vi "Func-엑셀 데이터를 그래프로 출력.vi"() -> ()   [LabVIEW 2015] (continued)
1252.26\n1252.28\n1252.29\n1252.31\n1252.33\n1252.34\n1252.36\n1252.38\n1252.39\n1252.41\n1252.43\n1252.44\n1252.46\n1252.48\n1252.49\n1252.51\n1252.53\n1252.54\n1252.56\n1252.58\n1252.59\n1252.61\n1252.63\n1252.64\n1252.66\n1252.68\n1252.69\n1252.71\n1252.73\n1252.74\n1252.76\n1252.78\n1252.79\n1252.81\n1252.83\n1252.84\n1252.86\n1252.88\n1252.89\n1252.91\n1252.93\n1252.94\n1252.96\n1252.98\n1252.99\n1253.01\n1253.03\n1253.04\n1253.06\n1253.08\n1253.09\n1253.11\n1253.13\n1253.14\n1253.16\n1253.18\n1253.2\n1253.21\n1253.23\n1253.24\n1253.26\n1253.28\n1253.3\n1253.31\n1253.33\n1253.34\n1253.36\n1253.38\n1253.39\n1253.41\n1253.43\n1253.44\n1253.46\n1253.48\n1253.49\n1253.51\n1253.53\n1253.55\n1253.56\n1253.58\n1253.59\n1253.61\n1253.63\n1253.64\n1253.66\n1253.68\n1253.69\n1253.71\n1253.73\n1253.74\n1253.76\n1253.78\n1253.79\n1253.81\n1253.83\n1253.84\n1253.86\n1253.88\n1253.9\n1253.91\n1253.93\n1253.94\n1253.96\n1253.98\n1253.99\n1254.01\n1254.03\n1254.04\n1254.06\n1254.08\n1254.09\n1254.11\n1254.13\n1254.14\n1254.16\n1254.18\n1254.19\n1254.21\n1254.23\n1254.25\n1254.26\n1254.28\n1254.29\n1254.31\n1254.33\n1254.35\n1254.36\n1254.38\n1254.39\n1254.41\n1254.43\n1254.44\n1254.46\n1254.48\n1254.5\n1254.51\n1254.53\n1254.54\n1254.56\n1254.58\n1254.59\n1254.61\n1254.63\n1254.64\n1254.66\n1254.68\n1254.69\n1254.71\n1254.73\n1254.74\n1254.76\n1254.78\n1254.79\n1254.81\n1254.83\n1254.84\n1254.86\n1254.88\n1254.89\n1254.91\n1254.93\n1254.94\n1254.96\n1254.98\n1254.99\n1255.01\n1255.03\n1255.04\n1255.06\n1255.08\n1255.09\n1255.11\n1255.13\n1255.15\n1255.16\n1255.18\n1255.19\n1255.21\n1255.23\n1255.24\n1255.26\n1255.28\n1255.29\n1255.31\n1255.33\n1255.34\n1255.36\n1255.38\n1255.39\n1255.41\n1255.43\n1255.44\n1255.46\n1255.48\n1255.49\n1255.51\n1255.53\n1255.54\n1255.56\n1255.58\n1255.59\n1255.61\n1255.63\n1255.64\n1255.66\n1255.68\n1255.69\n1255.71\n1255.73\n1255.74\n1255.76\n1255.78\n1255.79\n1255.81\n1255.83\n1255.84\n1255.86\n1255.88\n1255.89\n1255.91\n1255.93\n1255.95\n1255.96\n1255.98\n1255.99\n1256.01\n1256.03\n1256.04\n1256.06\n1256.08\n1256.09\n1256.11\n1256.13\n1256.14\n1256.16\n1256.18\n1256.19\n1256.21\n1256.23\n1256.24\n1256.26\n1256.28\n1256.3\n1256.31\n1256.33\n1256.34\n1256.36\n1256.38\n1256.39\n1256.41\n1256.43\n1256.44\n1256.46\n1256.48\n1256.49\n1256.51\n1256.53\n1256.54\n1256.56\n1256.58\n1256.59\n1256.61\n1256.63\n1256.65\n1256.66\n1256.68\n1256.69\n1256.71\n1256.73\n1256.74\n1256.76\n1256.78\n1256.79\n1256.81\n1256.83\n1256.85\n1256.86\n1256.88\n1256.9\n1256.91\n1256.93\n1256.94\n1256.96\n1256.98\n1257\n1257.01\n1257.03\n1257.04\n1257.06\n1257.08\n1257.09\n1257.11\n1257.13\n1257.14\n1257.16\n1257.18\n1257.2\n1257.21\n1257.23\n1257.25\n1257.26\n1257.28\n1257.29\n1257.31\n1257.33\n1257.35\n1257.36\n1257.38\n1257.39\n1257.41\n1257.43\n1257.45\n1257.46\n1257.48\n1257.49\n1257.51\n1257.53\n1257.54\n1257.56\n1257.58\n1257.6\n1257.61\n1257.63\n1257.64\n1257.66\n1257.68\n1257.69\n1257.71\n1257.73\n1257.74\n1257.76\n1257.78\n1257.79\n1257.81\n1257.83\n1257.84\n1257.86\n1257.88\n1257.89\n1257.91\n1257.93\n1257.94\n1257.96\n1257.98\n1257.99\n1258.01\n1258.03\n1258.04\n1258.06\n1258.08\n1258.09\n1258.11\n1258.13\n1258.14\n1258.16\n1258.18\n1258.19\n1258.21\n1258.23\n1258.24\n1258.26\n1258.28\n1258.29\n1258.31\n1258.33\n1258.35\n1258.36\n1258.38\n1258.39\n1258.41\n1258.43\n1258.44\n1258.46\n1258.48\n1258.49\n1258.51\n1258.53\n1258.54\n1258.56\n1258.58\n1258.59\n1258.61\n1258.63\n1258.64\n1258.66\n1258.68\n1258.69\n1258.71\n1258.73\n1258.74\n1258.76\n1258.78\n1258.79\n1258.81\n1258.83\n1258.85\n1258.86\n1258.88\n1258.89\n1258.91\n1258.93\n1258.94\n1258.96\n1258.98\n1258.99\n1259.01\n1259.03\n1259.05\n1259.06\n1259.08\n1259.09\n1259.11\n1259.13\n1259.14\n1259.16\n1259.18\n1259.19\n1259.21\n1259.23\n1259.24\n1259.26\n1259.28\n1259.3\n1259.31\n1259.33\n1259.34\n1259.36\n1259.38\n1259.4\n1259.41\n1259.43\n1259.44\n1259.46\n1259.48\n1259.49\n1259.51\n1259.53\n1259.54\n1259.56\n1259.58\n1259.59\n1259.61\n1259.63\n1259.65\n1259.66\n1259.68\n1259.69\n1259.71\n1259.73\n1259.75\n1259.76\n1259.78\n1259.8\n1259.81\n1259.83\n1259.85\n1259.86\n1259.88\n1259.89\n1259.91\n1259.93\n1259.94\n1259.96\n1259.98\n1260\n1260.01\n1260.03\n1260.04\n1260.06\n1260.08\n1260.09\n1260.11\n1260.13\n1260.14\n1260.16\n1260.18\n1260.19\n1260.21\n1260.23\n1260.24\n1260.26\n1260.28\n1260.29\n1260.31\n1260.33\n1260.34\n1260.36\n1260.38\n1260.39\n1260.41\n1260.43\n1260.44\n1260.46\n1260.48\n1260.49\n1260.51\n1260.53\n1260.54\n1260.56\n1260.58\n1260.59\n1260.61\n1260.63\n1260.65\n1260.66\n1260.68\n1260.69\n1260.71\n1260.73\n1260.74\n1260.76\n1260.78\n1260.79\n1260.81\n1260.83\n1260.84\n1260.86\n1260.88\n1260.89\n1260.91\n1260.93\n1260.94\n1260.96\n1260.98\n1260.99\n1261.01\n1261.03\n1261.04\n1261.06\n1261.08\n1261.09\n1261.11\n1261.13\n1261.14\n1261.16\n1261.18\n1261.19\n1261.21\n1261.23\n1261.24\n1261.26\n1261.28\n1261.29\n1261.31\n1261.33\n1261.34\n1261.36\n1261.38\n1261.39\n1261.41\n1261.43\n1261.44\n1261.46\n1261.48\n1261.49\n1261.51\n1261.53\n1261.54\n1261.56\n1261.58\n1261.59\n1261.61\n1261.63\n1261.64\n1261.66\n1261.68\n1261.69\n1261.71\n1261.73\n1261.74\n1261.76\n1261.78\n1261.79\n1261.81\n1261.83\n1261.84\n1261.86\n1261.88\n1261.89\n1261.91\n1261.93\n1261.94\n1261.96\n1261.98\n1261.99\n1262.01\n1262.03\n1262.05\n1262.06\n1262.08\n1262.09\n1262.11\n1262.13\n1262.15\n1262.16\n1262.18\n1262.19\n1262.21\n1262.23\n1262.24\n1262.26\n1262.28\n1262.29\n1262.31\n1262.33\n1262.34\n1262.36\n1262.38\n1262.39\n1262.41\n1262.43\n1262.44\n1262.46\n1262.48\n1262.5\n1262.51\n1262.53\n1262.55\n1262.56\n1262.58\n1262.6\n1262.61\n1262.63\n1262.64\n1262.66\n1262.68\n1262.69\n1262.71\n1262.73\n1262.75\n1262.76\n1262.78\n1262.79\n1262.81\n1262.83\n1262.85\n1262.86\n1262.88\n1262.89\n1262.91\n1262.93\n1262.94\n1262.96\n1262.98\n1262.99\n1263.01\n1263.03\n1263.04\n1263.06\n1263.08\n1263.1\n1263.11\n1263.13\n1263.14\n1263.16\n1263.18\n1263.19\n1263.21\n1263.23\n1263.24\n1263.26\n1263.28\n1263.29\n1263.31\n1263.33\n1263.35\n1263.36\n1263.38\n1263.39\n1263.41\n1263.43\n1263.45\n1263.46\n1263.48\n1263.5\n1263.51\n1263.53\n1263.54\n1263.56\n1263.58\n1263.59\n1263.61\n1263.63\n1263.64\n1263.66\n1263.68\n1263.69\n1263.71\n1263.73\n1263.74\n1263.76\n1263.78\n1263.79\n1263.81\n1263.83\n1263.84\n1263.86\n1263.88\n1263.89\n1263.91\n1263.93\n1263.94\n1263.96\n1263.98\n1263.99\n1264.01\n1264.03\n1264.04\n1264.06\n1264.08\n1264.09\n1264.11\n1264.13\n1264.14\n1264.16\n1264.18\n1264.19\n1264.21\n1264.23\n1264.24\n1264.26\n1264.28\n1264.29\n1264.31\n1264.33\n1264.34\n1264.36\n1264.38\n1264.39\n1264.41\n1264.43\n1264.44\n1264.46\n1264.48\n1264.49\n1264.51\n1264.53\n1264.55\n1264.56\n1264.58\n1264.59\n1264.61\n1264.63\n1264.64\n1264.66\n1264.68\n1264.69\n1264.71\n1264.73\n1264.74\n1264.76\n1264.78\n1264.79\n1264.81\n1264.83\n1264.84\n1264.86\n1264.88\n1264.89\n1264.91\n1264.93\n1264.94\n1264.96\n1264.98\n1264.99\n1265.01\n1265.03\n1265.04\n1265.06\n1265.08\n1265.09\n1265.11\n1265.13\n1265.14\n1265.16\n1265.18\n1265.19\n1265.21\n1265.23\n1265.25\n1265.26\n1265.28\n1265.29\n1265.31\n1265.33\n1265.34\n1265.36\n1265.38\n1265.39\n1265.41\n1265.43\n1265.44\n1265.46\n1265.48\n1265.5\n1265.51\n1265.53\n1265.54\n1265.56\n1265.58\n1265.6\n1265.61\n1265.63\n1265.64\n1265.66\n1265.68\n1265.69\n1265.71\n1265.73\n1265.75\n1265.76\n1265.78\n1265.79\n1265.81\n1265.83\n1265.85\n1265.86\n1265.88\n1265.89\n1265.91\n1265.93\n1265.95\n1265.96\n1265.98\n1265.99\n1266.01\n1266.03\n1266.04\n1266.06\n1266.08\n1266.09\n1266.11\n1266.13\n1266.14\n1266.16\n1266.18\n1266.19\n1266.21\n1283.85\n1283.86\n1283.9\n1283.93\n1283.96\n1284\n1284.03\n1284.06\n1284.1\n1284.13\n1284.16\n1284.2\n1284.23\n1284.26\n1284.3\n1284.33\n1284.36\n1284.4\n1284.43\n1284.46\n1284.49\n1284.53\n1284.56\n1284.59\n1284.63\n1284.66\n1284.7\n1284.73\n1284.76\n1284.8\n1284.83\n1284.86\n1284.9\n1284.93\n1284.96\n1284.99\n1285.03\n1285.06\n1285.09\n1285.13\n1285.16\n1285.2\n1285.23\n1285.26\n1285.3\n1285.33\n1285.36\n1285.4\n1285.43\n1285.46\n1285.5\n1285.53\n1285.56\n1285.6\n1285.63\n1285.66\n1285.7\n1285.73\n1285.76\n1285.79\n1285.83\n1285.86\n1285.9\n1285.93\n1285.96\n1286\n1286.03\n1286.06\n1286.1\n1286.13\n1286.16\n1286.2\n1286.23\n1286.26\n1286.3\n1286.33\n1286.36\n1286.4\n1286.43\n1286.46\n1286.5\n1286.53\n1286.56\n1286.6\n1286.63\n1286.66\n1286.7\n1286.73\n1286.76\n1286.8\n1286.83\n1286.86\n1286.9\n1286.93\n1286.96\n1287\n1287.03\n1287.06\n1287.1\n1287.13\n1287.16\n1287.2\n1287.23\n1287.26\n1287.3\n1287.33\n1287.36\n1287.39\n1287.43\n1287.46\n1287.49\n1287.53\n1287.56\n1287.59\n1287.63\n1287.66\n1287.71\n1287.73\n1287.76\n1287.8\n1287.83\n1287.86\n1287.9\n1287.93\n1287.96\n1288\n1288.03\n1288.06\n1288.09\n1288.13\n1288.16\n1288.19\n1288.23\n1288.26\n1288.3\n1288.33\n1288.36\n1288.4\n1288.43\n1288.46\n1288.5\n1288.53\n1288.56\n1288.6\n1288.63\n1288.66\n1288.7\n1288.73\n1288.76\n1288.8\n1288.83\n1288.86\n1288.89\n1288.93\n1288.96\n1289\n1289.03\n1289.06\n1289.1\n1289.13\n1289.16\n1289.2\n1289.23\n1289.26\n1289.3\n1289.33\n1289.36\n1289.4\n1289.43\n1289.46\n1289.5\n1289.53\n1289.56\n1289.6\n1289.63\n1289.66\n1289.7\n1289.73\n1289.76\n1289.8\n1289.83\n1289.86\n1289.9\n1289.93\n1289.96\n1290\n1290.03\n1290.06\n1290.1\n1290.13\n1290.16\n1290.2\n1290.23\n1290.26\n1290.3\n1290.33\n1290.36\n1290.39\n1290.43\n1290.46\n1290.49\n1290.53\n1290.56\n1290.6\n1290.63\n1290.66\n1290.69\n1290.75\n1290.76\n1290.8\n1290.83\n1290.86\n1290.9\n1290.93\n1290.96\n1291\n1291.03\n1291.06\n1291.1\n1291.13\n1291.16\n1291.19\n1291.23\n1291.26\n1291.29\n1291.35\n1291.36\n1291.4\n1291.43\n1291.46\n1291.5\n1291.53\n1291.56\n1291.6\n1291.63\n1291.66\n1291.7\n1291.73\n1291.76\n1291.8\n1291.83\n1291.86\n1291.9\n1291.95\n1291.96\n1292\n1292.03\n1292.06\n1292.1\n1292.13\n1292.16\n1292.2\n1292.23\n1292.26\n1292.3\n1292.33\n1292.36\n1292.4\n1292.43\n1292.46\n1292.5\n1292.55\n1292.56\n1292.6\n1292.63\n1292.66\n1292.7\n1292.73\n1292.76\n1292.8\n1292.83\n1292.86\n1292.9\n1292.93\n1292.96\n1293\n1293.03\n1293.06\n1293.1\n1293.15\n1293.16\n1293.2\n1293.23\n1293.26\n1293.3\n1293.33\n1293.36\n1293.4\n1293.43\n1293.46\n1293.49\n1293.53\n1293.56\n1293.6\n1293.63\n1293.66\n1293.71\n1293.73\n1293.76\n1293.8\n1293.83\n1293.86\n1293.9\n1293.93\n1293.96\n1294\n1294.03\n1294.06\n1294.1\n1294.13\n1294.16\n1294.2\n1294.23\n1294.26\n1294.29\n1294.33\n1294.36\n1294.39\n1294.43\n1294.46\n1294.5\n1294.53\n1294.56\n1294.6\n1294.63\n1294.66\n1294.7\n1294.73\n1294.76\n1294.8\n1294.83\n1294.86\n1294.9\n1294.95\n1294.96\n1294.99\n1295.03\n1295.06\n1295.1\n1295.13\n1295.16\n1295.2\n1295.23\n1295.26\n1295.3\n1295.33\n1295.36\n1295.4\n1295.43\n1295.46\n1295.5\n1295.53\n1295.58\n1295.61\n1295.63\n1295.66\n1295.7\n1295.73\n1295.76\n1295.8\n1295.83\n1295.86\n1295.9\n1295.93\n1295.96\n1296\n1296.03\n1296.06\n1296.1\n1296.13\n1296.18\n1296.2\n1296.23\n1296.26\n1296.3\n1296.33\n1296.36\n1296.4\n1296.43\n1296.46\n1296.5\n1296.53\n1296.56\n1296.6\n1296.63\n1296.66\n1296.7\n1296.73\n1296.76\n1296.81\n1296.83\n1296.86\n1296.89\n1296.93\n1296.96\n1297\n1297.03\n1297.06\n1297.1\n1297.13\n1297.16\n1297.2\n1297.23\n1297.26\n1297.3\n1297.33\n1297.36\n1297.39\n1297.43\n1297.46\n1297.49\n1297.53\n1297.56\n1297.6\n1297.63\n1297.66\n1297.7\n1297.73\n1297.76\n1297.8\n1297.83\n1297.86\n1297.9\n1297.93\n1297.98\n1298\n1298.03\n1298.06\n1298.1\n1298.13\n1298.16\n1298.2\n1298.23\n1298.26\n1298.3\n1298.33\n1298.36\n1298.4\n1298.43\n1298.46\n1298.5\n1298.53\n1298.56\n1298.61\n1298.65\n1298.66\n1298.7\n1298.73\n1298.76\n1298.8\n1298.83\n1298.86\n1298.9\n1298.93\n1298.96\n1299\n1299.03\n1299.06\n1299.1\n1299.13\n1299.16\n1299.2\n1299.23\n1299.26\n1299.3\n1299.33\n1299.36\n1299.4\n1299.43\n1299.46\n1299.5\n1299.53\n1299.56\n1299.6\n1299.63\n1299.66\n1299.7\n1299.73\n1299.76\n1299.79\n1299.85\n1299.86\n1299.89\n1299.93\n1299.96\n1300\n1300.03\n1300.06\n1300.1\n1300.13\n1300.16\n1300.2\n1300.23\n1300.26\n1300.3\n1300.33\n1300.36\n1300.41\n1300.43\n1300.46\n1300.49\n1300.53\n1300.56\n1300.6\n1300.63\n1300.66\n1300.7\n1300.73\n1300.77\n1300.78\n1300.79\n1300.79\n1300.8\n1300.81\n1300.82\n1300.83\n1300.84\n1300.84\n1300.85\n1300.86\n1300.87\n1300.88\n1300.89\n1300.89\n1300.9\n1300.91\n1300.92\n1300.93\n1300.94\n1300.94\n1300.95\n1300.96\n1300.97\n1300.98\n1300.99\n1300.99\n1301\n1301.01\n1301.02\n1301.03\n1301.04\n1301.04\n1301.05\n1301.06\n1301.07\n1301.08\n1301.09\n1301.09\n1301.1\n1301.11\n1301.12\n1301.13\n1301.14\n1301.14\n1301.15\n1301.16\n1301.17\n1301.18\n1301.19\n1301.19\n1301.2\n1301.21\n1301.22\n1301.23\n1301.24\n1301.24\n1301.25\n1301.26\n1301.27\n1301.28\n1301.29\n1301.29\n1301.3\n1301.31\n1301.32\n1301.33\n1301.34\n1301.34\n1301.35\n1301.36\n1301.37\n1301.38\n1301.39\n1301.39\n1301.4\n1301.41\n1301.42\n1301.43\n1301.44\n1301.44\n1301.45\n1301.46\n1301.47\n1301.48\n1301.49\n1301.49\n1301.5\n1301.51\n1301.52\n1301.53\n1301.54\n1301.55\n1301.55\n1301.56\n1301.57\n1301.58\n1301.59\n1301.59\n1301.6\n1301.61\n1301.62\n1301.63\n1301.64\n1301.64\n1301.65\n1301.66\n1301.67\n1301.68\n1301.69\n1301.69\n1301.7\n1301.71\n1301.72\n1301.73\n1301.74\n1301.74\n1301.75\n1301.76\n1301.77\n1301.78\n1301.79\n1301.79\n1301.8\n1301.81\n1301.82\n1301.83\n1301.84\n1301.84\n1301.85\n1301.86\n1301.87\n1301.88\n1301.89\n1301.9\n1301.9\n1301.91\n1301.92\n1301.93\n1301.94\n1301.94\n1301.95\n1301.96\n1301.97\n1301.98\n1301.99\n1302\n1302\n1302.01\n1302.02\n1302.03\n1302.04\n1302.04\n1302.05\n1302.06\n1302.07\n1302.08\n1302.09\n1302.09\n1302.1\n1302.11\n1302.12\n1302.13\n1302.14\n1302.15\n1302.15\n1302.16\n1302.17\n1302.18\n1302.19\n1302.19\n1302.2\n1302.21\n1302.22\n1302.23\n1302.24\n1302.25\n1302.25\n1302.26\n1302.27\n1302.28\n1302.29\n1302.29\n1302.3\n1302.31\n1302.32\n1302.33\n1302.34\n1302.35\n1302.35\n1302.36\n1302.37\n1302.38\n1302.39\n1302.39\n1302.4\n1302.41\n1302.42\n1302.43\n1302.44\n1302.44\n1302.45\n1302.46\n1302.47\n1302.48\n1302.49\n1302.5\n1302.5\n1302.51\n1302.52\n1302.53\n1302.54\n1302.54\n1302.55\n1302.56\n1302.57\n1302.58\n1302.59\n1302.6\n1302.6\n1302.61\n1302.62\n1302.63\n1302.64\n1302.64\n1302.65\n1302.66\n1302.67\n1302.68\n1302.69\n1302.7\n1302.7\n1302.71\n1302.72\n1302.73\n1302.74\n1302.74\n1302.75\n1302.76\n1302.77\n1302.78\n1302.79\n1302.79\n1302.8\n1302.81\n1302.82\n1302.83\n1302.84\n1302.84\n1302.85\n1302.86\n1302.87\n1302.88\n1302.89\n1302.89\n1302.9\n1302.91\n1302.92\n1302.93\n1302.94\n1302.94\n1302.95\n1302.96\n1302.97\n1302.98\n1302.99\n1302.99\n1303\n1303.01\n1303.02\n1303.03\n1303.04\n1303.04\n1303.05\n1303.06\n1303.07\n1303.08\n1303.09\n1303.09\n1303.1\n1303.11\n1303.12\n1303.13\n1303.14\n1303.14\n1303.15\n1303.16\n1303.17\n1303.18\n1303.19\n1303.19\n1303.2\n1303.21\n1303.22\n1303.23\n1303.24\n1303.24\n1303.25\n1303.26\n1303.27\n1303.28\n1303.29\n1303.29\n1303.3\n1303.31\n1303.32\n1303.33\n1303.34\n1303.34\n1303.35\n1303.36\n1303.37\n1303.38\n1303.39\n1303.39\n1303.4\n1303.41\n1303.42\n1303.43\n1303.44\n1303.44\n1303.45\n1303.46\n1303.47\n1303.48\n1303.49\n1303.49\n1303.5\n1303.51\n1303.52\n1303.53\n1303.54\n1303.54\n1303.55\n1303.56\n1303.57\n1303.58\n1303.59\n1303.59\n1303.6\n1303.61\n1303.62\n1303.63\n1303.64\n1303.64\n1303.65\n1303.66\n1303.67\n1303.68\n1303.69\n1303.69\n1303.7\n1303.71\n1303.72\n1303.73\n1303.74\n1303.74\n1303.75\n1303.76\n1303.77\n1303.78\n1303.79\n1303.79\n1303.8\n1303.81\n1303.82\n1303.83\n1303.84\n1303.84\n1303.85\n1303.86\n1303.87\n1303.88\n1303.89\n1303.89\n1303.9\n1303.91\n1303.92\n1303.93\n1303.94\n1303.94\n1303.95\n1303.96\n1303.97\n1303.98\n1303.99\n1303.99\n1304\n1304.01\n1304.02\n1304.03\n1304.04\n1304.04\n1304.05\n1304.06\n1304.07\n1304.08\n1304.09\n1304.09\n1304.1\n1304.11\n1304.12\n1304.13\n1304.14\n1304.14\n1304.15\n1304.16\n1304.17\n1304.18\n1304.19\n1304.19\n1304.2\n1304.21\n1304.22\n1304.23\n1304.24\n1304.24\n1304.25\n1304.26\n1304.27\n1304.28\n1304.29\n1304.3\n1304.3\n1304.31\n1304.32\n1304.33\n1304.34\n1304.34\n1304.35\n1304.36\n1304.37\n1304.38\n1304.39\n1304.39\n1304.4\n1304.41\n1304.42\n1304.43\n1304.44\n1304.44\n1304.45\n1304.46\n1304.47\n1304.48\n1304.49\n1304.49\n1304.5\n1304.51\n1304.52\n1304.53\n1304.54\n1304.54\n1304.55\n1304.56\n1304.57\n1304.58\n1304.59\n1304.59\n1304.6\n1304.61\n1304.62\n1304.63\n1304.64\n1304.64\n1304.65\n1304.66\n1304.67\n1304.68\n1304.69\n1304.69\n1304.7\n1304.71\n1304.72\n1304.73\n1304.74\n1304.74\n1304.75\n1304.76\n1304.77\n1304.78\n1304.79\n1304.79\n1304.8\n1304.81\n1304.82\n1304.83\n1304.84\n1304.84\n1304.85\n1304.86\n1304.87\n1304.88\n1304.89\n1304.89\n1304.9\n1304.91\n1304.92\n1304.93\n1304.94\n1304.94\n1304.95\n1304.96\n1304.97\n1304.98\n1304.99\n1305\n1305\n1305.01\n1305.02\n1305.03\n1305.04\n1305.04\n1305.05\n1305.06\n1305.07\n1305.08\n1305.09\n1305.09\n1305.1\n1305.11\n1305.12\n1305.13\n1305.14\n1305.14\n1305.15\n1305.16\n1305.17\n1305.18\n1305.19\n1305.19\n1305.2\n1305.21\n1305.22\n1305.23\n1305.24\n1305.25\n1305.25\n1305.26\n1305.27\n1305.28\n1305.29\n1305.29\n1305.3\n1305.31\n1305.32\n1305.33\n1305.34\n1305.35\n1305.35\n1305.36\n1305.37\n1305.38\n1305.39\n1305.39\n1305.4\n1305.41\n1305.42\n1305.43\n1305.44\n1305.44\n1305.45\n1305.46\n1305.47\n1305.48\n1305.49\n1305.49\n1305.5\n1305.51\n1305.52\n1305.53\n1305.54\n1305.54\n1305.55\n1305.56\n1305.57\n1305.58\n1305.59\n1305.6\n1305.6\n1305.61\n1305.62\n1305.63\n1305.64\n1305.64\n1305.65\n1305.66\n1305.67\n1305.68\n1305.69\n1305.7\n1305.7\n1305.71\n1305.72\n1305.73\n1305.74\n1305.74\n1305.75\n1305.77\n"
  in  "Y축 1":string="DPS 센서 전압(V)\n0.0003128\n0.00400914\n0.04822016\n0.09243478\n0.13661741\n0.18088003\n0.22513907\n0.26934129\n0.31354249\n0.35775453\n0.40194234\n0.44613013\n0.49034372\n0.53449279\n0.57871258\n0.62287194\n0.6670804\n0.71124184\n0.755328\n0.79956377\n0.84357244\n0.88760281\n0.93174618\n0.97576469\n1.01980484\n1.06384337\n1.10792947\n1.15197122\n1.19586015\n1.23986363\n1.28386247\n1.28381348\n1.24059355\n1.19588339\n1.15184271\n1.10791147\n1.06387436\n1.0198667\n0.97577345\n0.93180454\n0.88765496\n0.84360033\n0.79950494\n0.75538582\n0.71119487\n0.6671325\n0.62288386\n0.57876468\n0.53458673\n0.49045056\n0.44623077\n0.40202236\n0.35782215\n0.31363541\n0.26943782\n0.22521442\n0.18101114\n0.13677071\n0.09252615\n0.048247\n0.00409276\n0.00031384\n"
  # "엑셀 데이터를 그래프로 출력한다\n>> 열헤더 문자열 포함. (첫 라인)"
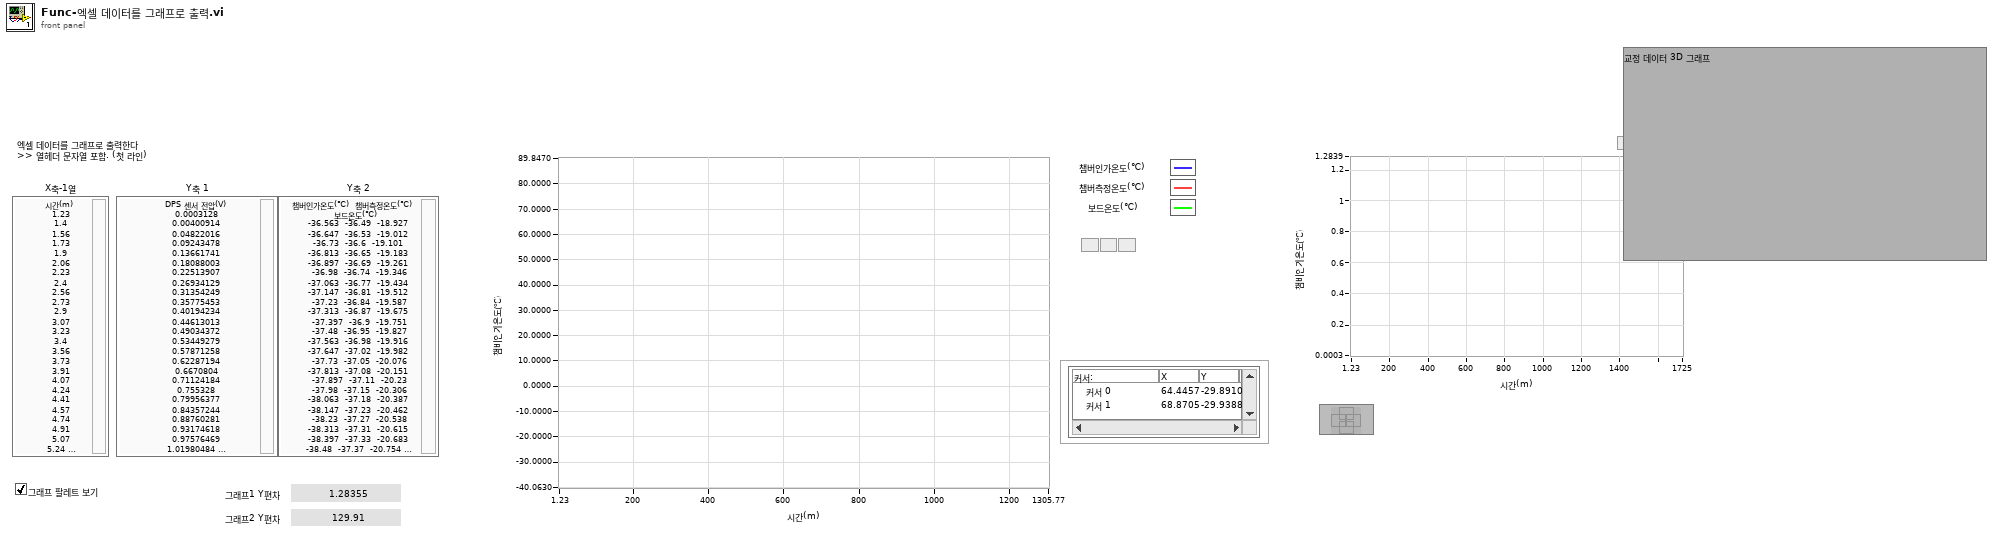
[diagram p1: front panel]
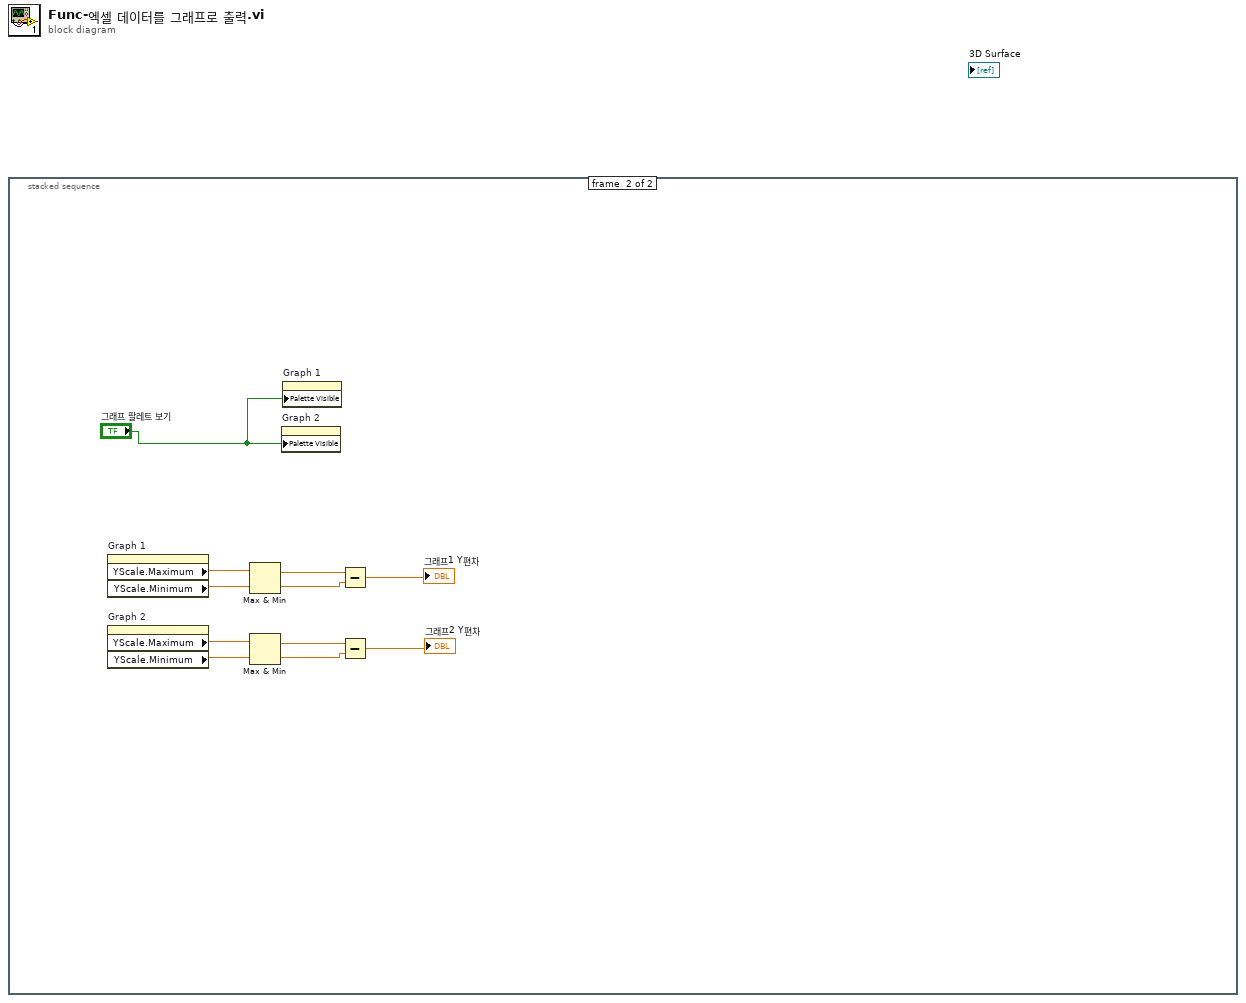
[diagram p0: block diagram]
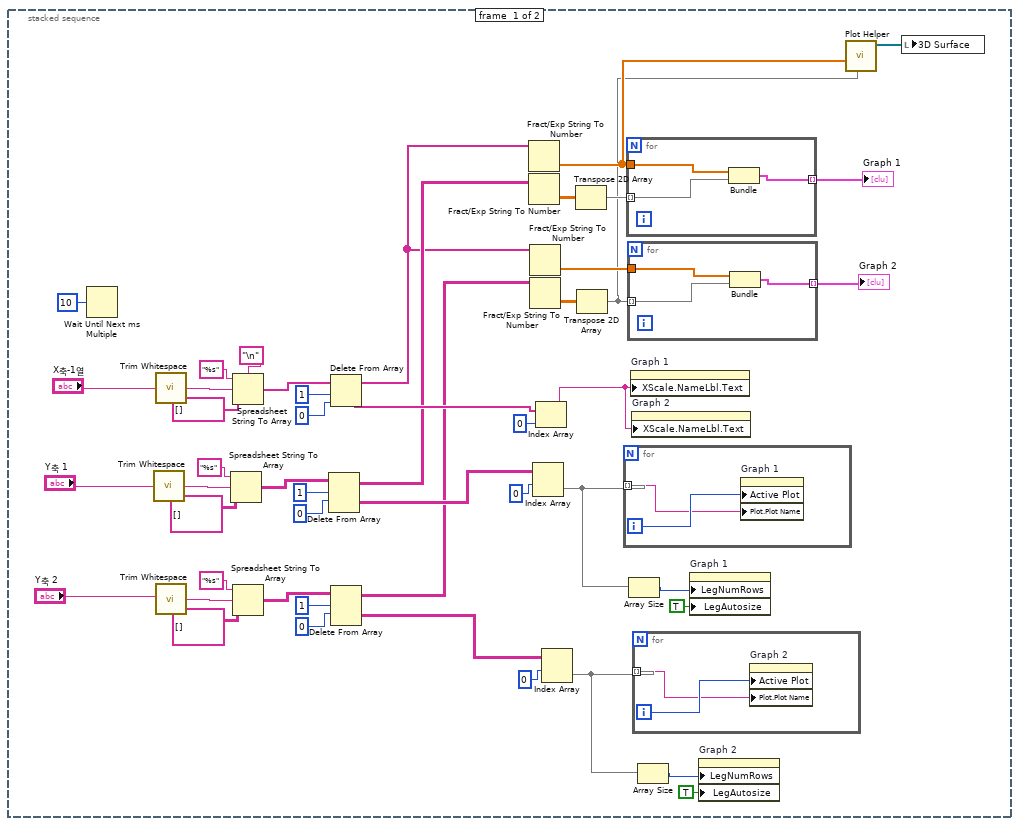
[diagram p2: hidden frame]
diagram:
  n1 = stacked-sequence {
    frame #0 {
      n2 = Wait Until Next ms Multiple(millisecond multiple=u32 10 ("ms 배수")) -> ()  [unwired: 1 out]
      n3 = call <vilib>:"Trim Whitespace.vi"("string"="Y축 1") -> ("trimmed string"=w35:string)  [unwired: 1 in]
      n4 = call <vilib>:"Trim Whitespace.vi"("string"="X축-1열") -> ("trimmed string"=w46:string)  [unwired: 1 in]
      n5 = call <vilib>:"Trim Whitespace.vi"("string"="Y축 2") -> ("trimmed string"=w18:string)  [unwired: 1 in]
      n6 = Spreadsheet String To Array(format string="%s" ("스프레드시트 문자열"), spreadsheet string=w35, array type (2D Dbl)=string[][] [] ("배열 타입(2D Dbl)")) -> (array=w36:string[][])  [unwired: 1 in]
      n7 = Spreadsheet String To Array(delimiter (Tab)="\n" ("스프레드시트 문자열"), format string="%s" ("스프레드시트 문자열"), spreadsheet string=w46, array type (2D Dbl)=string[] [] ("배열 타입(2D Dbl)")) -> (array=w43:string[])
      n8 = Spreadsheet String To Array(format string="%s" ("스프레드시트 문자열"), spreadsheet string=w18, array type (2D Dbl)=string[][] [] ("배열 타입(2D Dbl)")) -> (array=w17:string[][])  [unwired: 1 in]
      n9 = Delete From Array(array=w36, length=1 ("길이"), index (row)=0 ("길이")) -> (deleted portion=w29:string[][], array with subset deleted=w22:string[][])  [unwired: 1 in]
      n10 = Delete From Array(array=w43, length=1 ("길이"), index=0 ("길이")) -> (deleted portion=w39:string[], array with subset deleted=w12:string[])
      n11 = Delete From Array(array=w17, length=1 ("길이"), index (row)=0 ("길이")) -> (deleted portion=w6:string[][], array with subset deleted=w11:string[][])  [unwired: 1 in]
      n12 = Fract/Exp String To Number(string=w12) -> (number=w3:dbl[])  [unwired: 3 in, 1 out]
      n13 = Fract/Exp String To Number(string=w22) -> (number=w27:dbl[][])  [unwired: 3 in, 1 out]
      n14 = Fract/Exp String To Number(string=w12) -> (number=w14:dbl[])  [unwired: 3 in, 1 out]
      n15 = Fract/Exp String To Number(string=w11) -> (number=w2:dbl[][])  [unwired: 3 in, 1 out]
      n16 = Index Array(array=w29, index (row)=0 ("인덱스")) -> (element=w24:string[])  [unwired: 1 in]
      n17 = Index Array(array=w39, index=0 ("인덱스")) -> (element=w5:string)
      n18 = Index Array(array=w6, index (row)=0 ("인덱스")) -> (element=w9:string[])  [unwired: 1 in]
      n19 = Transpose 2D Array(2D array=w27) -> (transposed array=w26:dbl[][])
      n20 = Transpose 2D Array(2D array=w2) -> (transposed array=w1:dbl[][])
      n21 = for {
        tunnel: w24 -> [w57] mode=indexing
        i -> [w58]
        n22 = property on="Graph 1" class="XYGraph (엄격한)"("Active Plot"=w58, "Plot.Plot Name"=w57) -> ()  [unwired: 2 in, 2 out]
      }
      n23 = for {
        tunnel: w3 -> [w56]
        tunnel: w26 -> [w55] mode=indexing
        tunnel: [w54] -> w28 mode=indexing
        n24 = Bundle(w56, w55) -> (w54:cluster{dbl[], dbl[]})  [unwired: 1 in]
      }
      "Graph 1" <- w28
      n25 = for {
        tunnel: w14 -> [w53]
        tunnel: w1 -> [w52] mode=indexing
        tunnel: [w51] -> w13 mode=indexing
        n26 = Bundle(w53, w52) -> (w51:cluster{dbl[], dbl[]})  [unwired: 1 in]
      }
      "Graph 2" <- w13
      n27 = Array Size(array=w24) -> (size(s)=w23:i32)
      n28 = property on="Graph 1" class="XYGraph (엄격한)"("XScale.NameLbl.Text"=w5) -> ()  [unwired: 2 in, 2 out]
      n29 = property on="Graph 2" class="XYGraph (엄격한)"("XScale.NameLbl.Text"=w5) -> ()  [unwired: 2 in, 2 out]
      n30 = for {
        tunnel: w9 -> [w49] mode=indexing
        i -> [w50]
        n31 = property on="Graph 2" class="XYGraph (엄격한)"("Active Plot"=w50, "Plot.Plot Name"=w49) -> ()  [unwired: 2 in, 2 out]
      }
      n32 = Array Size(array=w9) -> (size(s)=w10:i32)
      n33 = property on="Graph 1" class="XYGraph (엄격한)"("LegNumRows"=w23, "LegAutosize"=TRUE ("범례:자동 크기 조정")) -> ()  [unwired: 2 in, 2 out]
      n34 = property on="Graph 2" class="XYGraph (엄격한)"("LegNumRows"=w10, "LegAutosize"=TRUE ("범례:자동 크기 조정")) -> ()  [unwired: 2 in, 2 out]
      n35 = call-poly <vilib>:"Plot Helper.vi"("z matrix"=w1, "y vector"=w3) -> ("3D Plot lvclass Array out"=w4:refnum<class "3D Plot Datatype.lvclass">[])  [unwired: 4 in, 5 out]
      n36 = local write "3D Surface"(w4) -> ()
    }
    frame #1 {
      n37 = property on="Graph 1" class="XYGraph (엄격한)"() -> ("YScale.Maximum"=w67:dbl, "YScale.Minimum"=w68:dbl)  [unwired: 2 in, 2 out]
      n38 = property on="Graph 2" class="XYGraph (엄격한)"() -> ("YScale.Maximum"=w61:dbl, "YScale.Minimum"=w60:dbl)  [unwired: 2 in, 2 out]
      n39 = Max & Min(x=w67, y=w68) -> (max(x,y)=w66:dbl, min(x,y)=w65:dbl)
      n40 = Max & Min(x=w61, y=w60) -> (max(x,y)=w62:dbl, min(x,y)=w63:dbl)
      n41 = property on="Graph 2" class="XYGraph (엄격한)"("Palette Visible"="그래프 팔레트 보기") -> ()  [unwired: 2 in, 2 out]
      n42 = property on="Graph 1" class="XYGraph (엄격한)"("Palette Visible"="그래프 팔레트 보기") -> ()  [unwired: 2 in, 2 out]
      n43 = Subtract(x=w66, y=w65) -> (x-y=→"그래프1 Y편차":dbl)
      n44 = Subtract(x=w62, y=w63) -> (x-y=→"그래프2 Y편차":dbl)
    }
  }
